vi "Test.vi"() -> ()   [LabVIEW 2012, in "Generic Data Logger.lvlib"]
uses:
  Generic Data Logger.lvlib
  Fluke 2625A (Hydra II)/Fluke 2625A (Hydra II).lvclass
  <vilib>/ActorFramework/Message Queue/Message Queue.lvclass/Message Queue.ctl
  <vilib>/ActorFramework/Message Enqueuer/Message Enqueuer.lvclass/Message Enqueuer.ctl
  <vilib>/ActorFramework/Message Enqueuer/Enqueue.vi
  <vilib>/ActorFramework/Message Priority Queue/Priority Enqueue.vi
  <vilib>/ActorFramework/Stop Msg/Stop Msg.lvclass
  Generic Instrument/Generic Instrument.lvclass
  Generic Data Logger.lvclass
  <vilib>/ActorFramework/Message Queue/Message Queue.lvclass
  <vilib>/ActorFramework/Actor/Actor.lvclass
panel:
  in  "Stop Button":bool
  out "error out":errorcluster
  in  "VISA resource name":refnum<visa-resource-name>
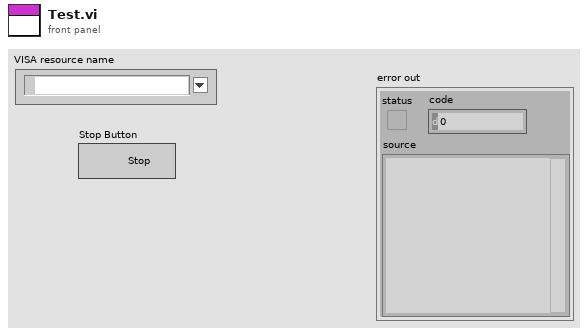
[diagram p1: front panel]
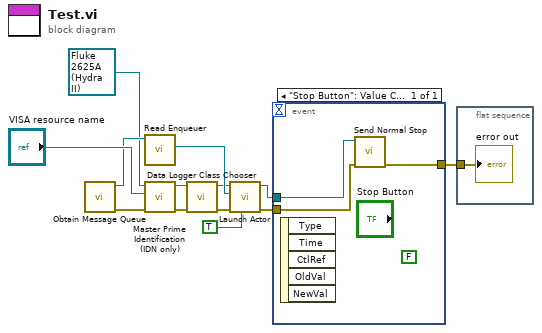
[diagram p0: block diagram]
diagram:
  n1 = call <vilib>:"Obtain Message Queue.vi"() -> ("error out"=w8:errorcluster, "Message Queue"=w9:refnum<class "Message Queue.lvclass">)  [unwired: 10 in]
  n2 = call <vilib>:"Read Enqueuer.vi"("Message Queue"=w9) -> ("Message Enqueuer"=w7:refnum<class "Message Enqueuer.lvclass">)  [unwired: 10 in]
  n3 = call "Master Prime Identification (IDN only).vi"("error in (no error)"=w8, "VISA resource name"="VISA resource name", "Generic Instrument.lvlib:Generic Instrument.lvclass"=refnum<class "Fluke 2625A (Hydra II).lvclass"> refnum ("Generic Data Logger.lvlib:Fluke 2625A (Hydra II).lvlib:Fluke 2625A (Hydra II).lvclass")) -> ("error out"=w11:errorcluster, "Generic Instrument out"=w12:refnum<class "Fluke 2625A (Hydra II).lvclass">)  [unwired: 7 in]
  n4 = call "Data Logger Class Chooser.vi"("error in (no error)"=w11, "Generic Instrument.lvlib:Generic Instrument.lvclass"=w12) -> ("error out"=w5:errorcluster, "Generic Instrument out"=w6:refnum<class "Fluke 2625A (Hydra II).lvclass">)  [unwired: 8 in]
  n5 = call <vilib>:"Launch Actor.vi"("Open Actor Core front panel? (F)"=TRUE, "error in (no error)"=w5, "Actor-to-Caller Enqueuer"=w7, "Actor"=w6) -> ("error out"=w1:errorcluster, "Caller-To-Actor Enqueuer"=w2:refnum<class "Message Enqueuer.lvclass">)  [unwired: 6 in]
  n6 = event shown="[0] \"Stop Button\": Value Change" {
    selector: _ -> [_]
    dyn-events: _ -> [_]
    timeout: _ -> [_]
    tunnel: w2 -> [w14]
    tunnel: w1 -> [w16]
    tunnel: [w15] -> w3
    event "Stop Button": Value Change {
      (unwired) FALSE ("Start/Stop")
      n7 = event-data() -> ()  [unwired: 1 in, 5 out]
      n8 = call <vilib>:"Send Normal Stop.vi"("error in (no error)"=w16, "Message Enqueuer"=w14) -> ("error out"=w15:errorcluster)  [unwired: 9 in]
    }
  }
  n9 = flat-sequence {
    tunnel: w3 -> [w17]
    frame #0 {
      "error out" <- w17
    }
  }
